vi "Ando Control.vi"() -> ()   [LabVIEW 2011]
panel:
  in  "Display Trace C":bool=TRUE
  in  "Trace C":enum16{"Fix", "Write"}(ring)=3
  in  "Display Trace B":bool=TRUE
  in  "Trace B":enum16{"Fix", "Write"}(ring)=3
  out "error out":errorcluster
  in  "Display Trace A":bool=TRUE
  in  "Trace A":enum16{"Fix", "Write"}(ring)=3
  in  "?":bool
  in  "?":bool
  in  "Log Scale dB/D (5)":dbl=10.0 min=0.1 max=10.0 step=0.1 format="%.1f"
  in  "Ref Level dBm (0)":dbl=-20.0 min=-90.0 max=20.0 step=0.1 format="%.1f"
  in  "Resolution (7: 2.0 nm)":T1(ring)
  in  "Sens (5:Norm Hold)":T2(ring)=enum."Norm Auto"
  in  "VISA session":refnum<visa-resource-name>="GPIB0::1::INSTR"
  in  "Span (1000 nm) 5":dbl=100.0 min=0.0 max=1200.0 step=0.1 format="%.2f"
  in  "Center (1250 nm) 5":dbl=1550.0 min=600.0 max=1750.0 step=0.01 format="%.2f"
  in  "Stop":bool
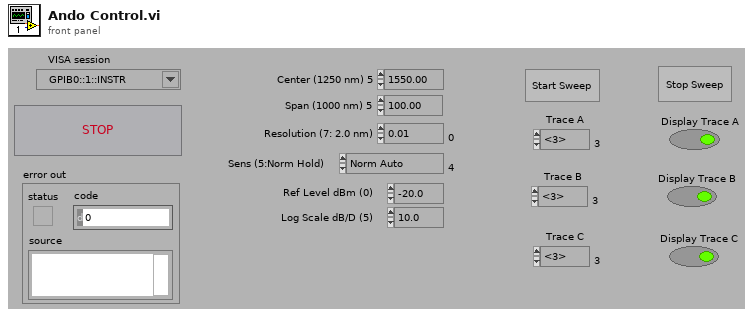
[diagram p1: front panel]
types:
  T1 = enum16{"0.01", "0.02", "0.05", "0.1", "0.2", "0.5", "1.0", "2.0"}
  T2 = enum16{"High 3", "High 2", "High 1", "Mid", "Norm Auto", "Norm Hold"}
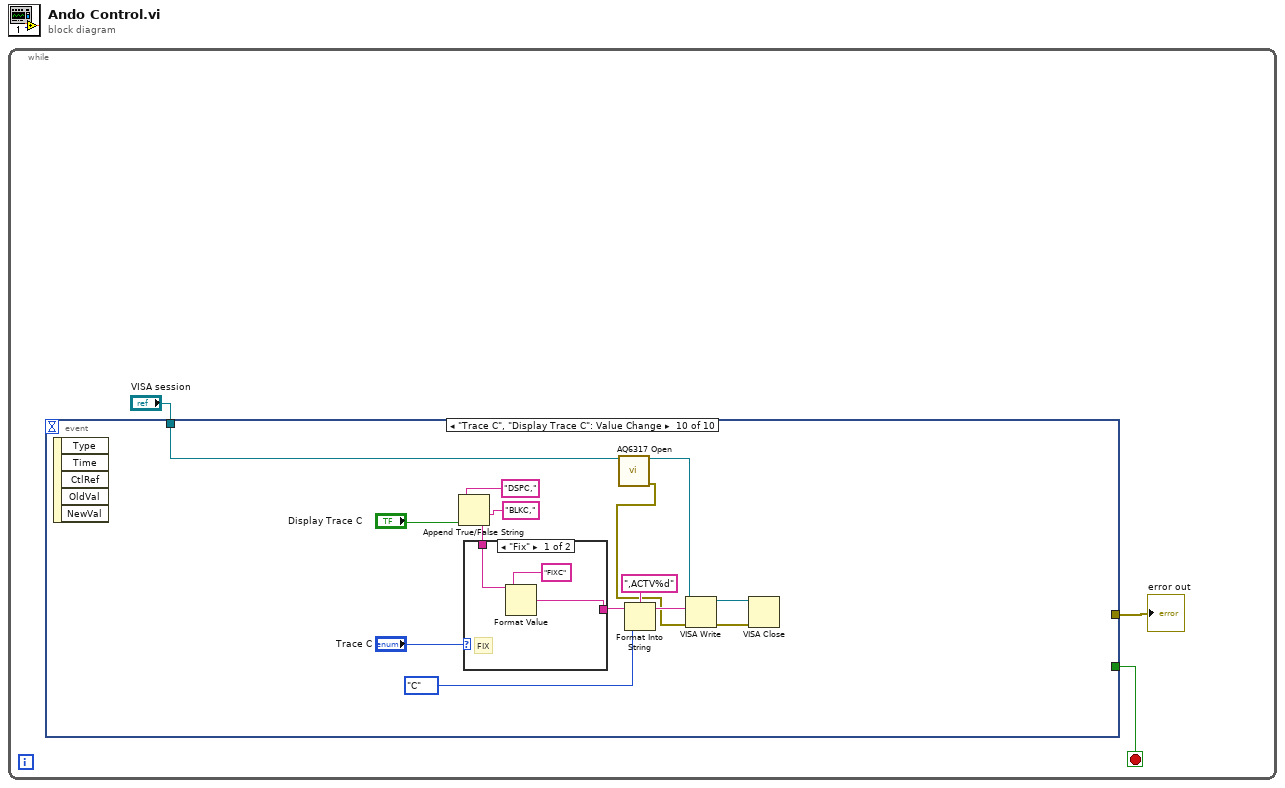
[diagram p0: block diagram]
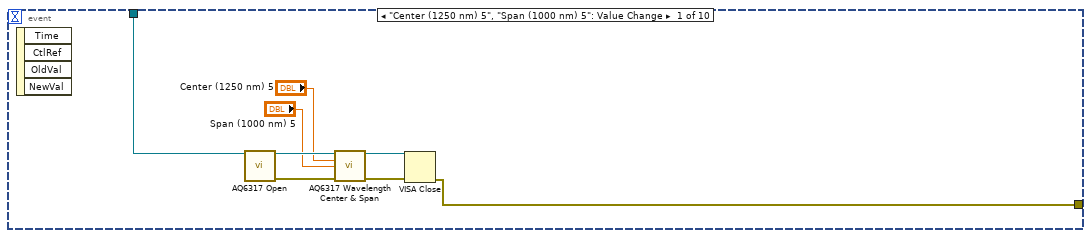
[diagram p2: hidden frame]
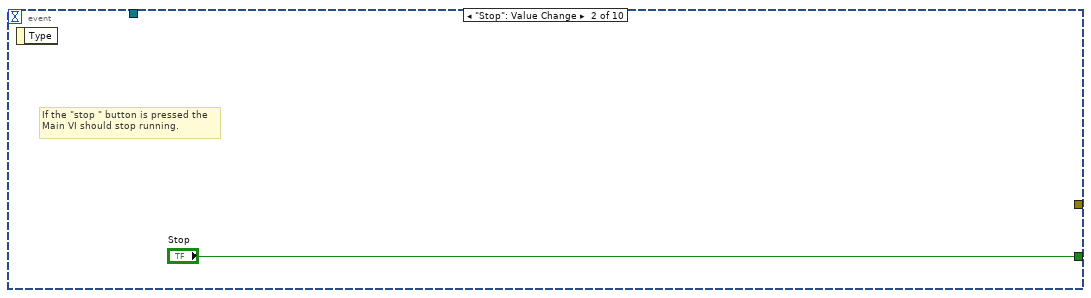
[diagram p3: hidden frame]
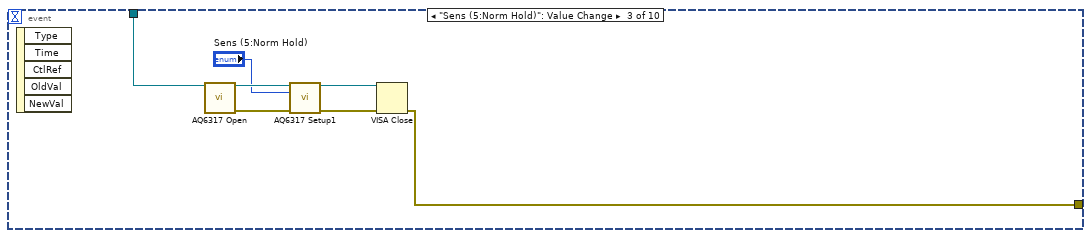
[diagram p4: hidden frame]
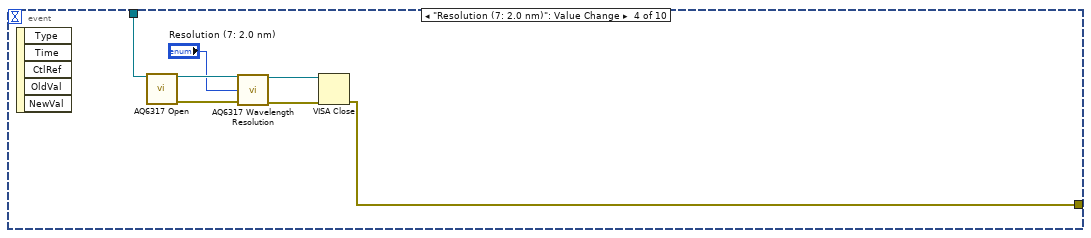
[diagram p5: hidden frame]
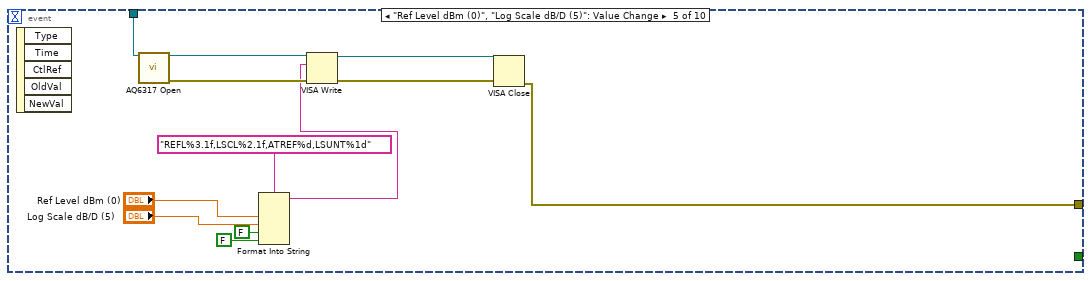
[diagram p6: hidden frame]
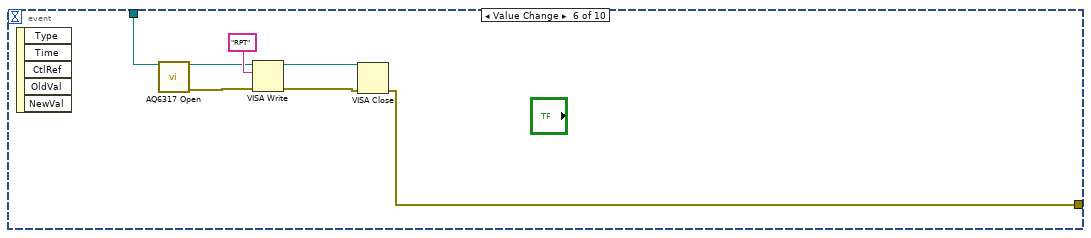
[diagram p7: hidden frame]
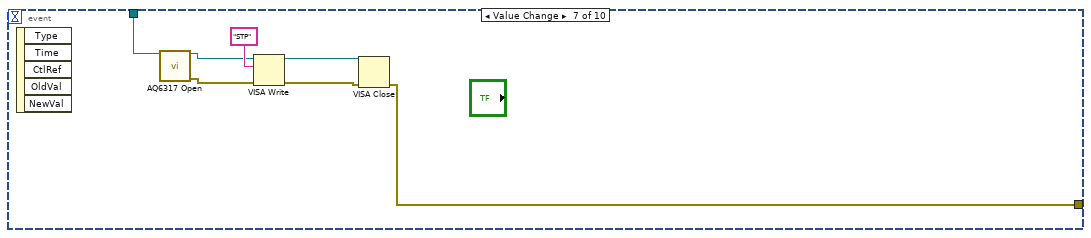
[diagram p8: hidden frame]
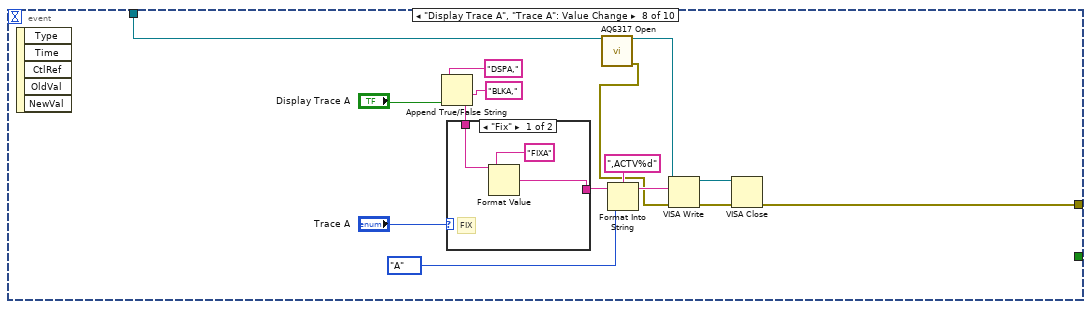
[diagram p9: hidden frame]
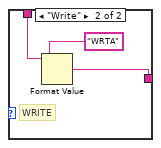
[diagram p10: hidden frame]
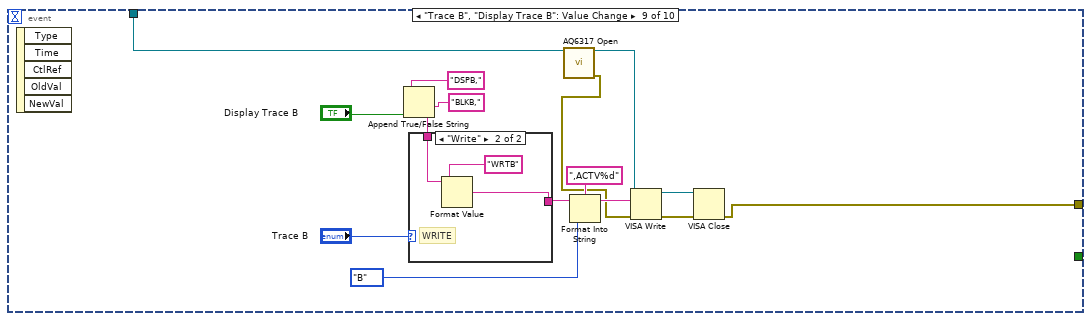
[diagram p11: hidden frame]
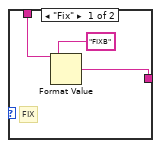
[diagram p12: hidden frame]
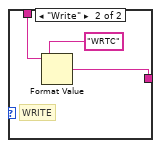
[diagram p13: hidden frame]
diagram:
  n1 = while {
    stop <- w3 stop-if-true
    n2 = event shown="[9] \"Trace C\", \"Display Trace C\": Value Change" {
      selector: _ -> [_ _ _ _ _ _ _ _ _ _]
      dyn-events: _ -> [_ _ _ _ _ _ _ _ _ _]
      timeout: _ -> [_ _ _ _ _ _ _ _ _ _]
      tunnel: [_ "Stop" _ _ _ _ _ _ _ _] -> w3
      tunnel: "VISA session" -> [w7 _ w19 w26 w36 w40 w51 w58 w75 w95]
      tunnel: [w4 _ w13 w20 w27 w39 w46 w53 w74 _] -> w1
      event "Center (1250 nm) 5", "Span (1000 nm) 5": Value Change {
        n3 = event-data() -> ()  [unwired: 5 out]
        n4 = call <instrlib>:"AQ6317 Open.vi"("VISA session (for class)"=w7) -> ("VISA session out"=w11:refnum<visa-resource-name>, "Error Out"=w10:errorcluster)  [unwired: 13 in]
        n5 = call <instrlib>:"AQ6317 Wavelength Center & Span.vi"("VISA session"=w11, "Center (1250 nm)"="Center (1250 nm) 5", "Span (1000 nm)"="Span (1000 nm) 5", "Error In"=w10) -> ("dup VISA session"=w9:refnum<visa-resource-name>, "Error Out"=w8:errorcluster)  [unwired: 10 in]
        n6 = VISA Close(VISA resource name=w9, error in (no error)=w8) -> (error out=w4:errorcluster)
      }
      event "Stop": Value Change {
        # "If the \"stop \" button is pressed the\nMain VI should stop running."
        n7 = event-data() -> ()  [unwired: 2 out]
      }
      event "Sens (5:Norm Hold)": Value Change {
        n8 = event-data() -> ()  [unwired: 6 out]
        n9 = call <instrlib>:"AQ6317 Open.vi"("VISA session (for class)"=w19) -> ("VISA session out"=w18:refnum<visa-resource-name>, "Error Out"=w17:errorcluster)  [unwired: 13 in]
        n10 = call <instrlib>:"AQ6317 Setup1.vi"("VISA session"=w18, "Sens (5:Norm Hold)"="Sens (5:Norm Hold)", "Error In"=w17) -> ("dup VISA session"=w15:refnum<visa-resource-name>, "Error Out"=w16:errorcluster)  [unwired: 11 in]
        n11 = VISA Close(VISA resource name=w15, error in (no error)=w16) -> (error out=w13:errorcluster)
      }
      event "Resolution (7: 2.0 nm)": Value Change {
        n12 = event-data() -> ()  [unwired: 6 out]
        n13 = call <instrlib>:"AQ6317 Open.vi"("VISA session (for class)"=w26) -> ("VISA session out"=w25:refnum<visa-resource-name>, "Error Out"=w23:errorcluster)  [unwired: 13 in]
        n14 = call <instrlib>:"AQ6317 Wavelength Resolution.vi"("VISA session"=w25, "Resolution (7: 2.0 nm)"="Resolution (7: 2.0 nm)", "Error In"=w23) -> ("dup VISA session"=w24:refnum<visa-resource-name>, "Error Out"=w22:errorcluster)  [unwired: 11 in]
        n15 = VISA Close(VISA resource name=w24, error in (no error)=w22) -> (error out=w20:errorcluster)
      }
      event "Ref Level dBm (0)", "Log Scale dB/D (5)": Value Change {
        n16 = event-data() -> ()  [unwired: 6 out]
        n17 = call <instrlib>:"AQ6317 Open.vi"("VISA session (for class)"=w36) -> ("VISA session out"=w35:refnum<visa-resource-name>, "Error Out"=w34:errorcluster)  [unwired: 13 in]
        n18 = Format Into String(format string="REFL%3.1f,LSCL%2.1f,ATREF%d,LSUNT%1d", "Ref Level dBm (0)", "Log Scale dB/D (5)", FALSE ("input 3"), FALSE ("input 4")) -> (resulting string=w28:string)  [unwired: 2 in, 1 out]
        n19 = VISA Write(VISA resource name=w35, write buffer=w28, error in (no error)=w34) -> (VISA resource name out=w37:refnum<visa-resource-name>, error out=w38:errorcluster)  [unwired: 1 out]
        n20 = VISA Close(VISA resource name=w37, error in (no error)=w38) -> (error out=w27:errorcluster)
      }
      event Value Change {
        n21 = event-data() -> ()  [unwired: 6 out]
        n22 = call <instrlib>:"AQ6317 Open.vi"("VISA session (for class)"=w40) -> ("VISA session out"=w44:refnum<visa-resource-name>, "Error Out"=w42:errorcluster)  [unwired: 13 in]
        n23 = VISA Write(VISA resource name=w44, write buffer="RPT", error in (no error)=w42) -> (VISA resource name out=w43:refnum<visa-resource-name>, error out=w41:errorcluster)  [unwired: 1 out]
        n24 = VISA Close(VISA resource name=w43, error in (no error)=w41) -> (error out=w39:errorcluster)
      }
      event Value Change {
        n25 = event-data() -> ()  [unwired: 6 out]
        n26 = call <instrlib>:"AQ6317 Open.vi"("VISA session (for class)"=w51) -> ("VISA session out"=w50:refnum<visa-resource-name>, "Error Out"=w48:errorcluster)  [unwired: 13 in]
        n27 = VISA Write(VISA resource name=w50, write buffer="STP", error in (no error)=w48) -> (VISA resource name out=w49:refnum<visa-resource-name>, error out=w47:errorcluster)  [unwired: 1 out]
        n28 = VISA Close(VISA resource name=w49, error in (no error)=w47) -> (error out=w46:errorcluster)
      }
      event "Display Trace A", "Trace A": Value Change {
        n29 = event-data() -> ()  [unwired: 6 out]
        n30 = Append True/False String(1:"Display Trace A", 2:"BLKA," ("false string"), 3:"DSPA," ("true string")) -> (0:w64:string)  [unwired: 1 in]
        n31 = case shown="\"Fix\"" "Trace A" {
          tunnel: w64 -> [w69 w72]
          tunnel: [w68 w71] -> w61
          frame "Fix" {
            # "FIX"
            n32 = Format Value(string ("")=w69, format string="FIXA") -> (output string=w68:string)  [unwired: 1 in]
          }
          frame "Write" {
            # "WRITE"
            n33 = Format Value(string ("")=w72, format string="WRTA") -> (output string=w71:string)  [unwired: 1 in]
          }
        }
        n34 = call <instrlib>:"AQ6317 Open.vi"("VISA session (for class)"=w58) -> ("VISA session out"=w57:refnum<visa-resource-name>, "Error Out"=w56:errorcluster)  [unwired: 13 in]
        n35 = Format Into String(format string=",ACTV%d", initial string=w61, enum16{"A", "B", "C"}."A" ("Active Trace (0:A)")) -> (resulting string=w60:string)  [unwired: 1 in, 1 out]
        n36 = VISA Write(VISA resource name=w57, write buffer=w60, error in (no error)=w56) -> (VISA resource name out=w55:refnum<visa-resource-name>, error out=w54:errorcluster)  [unwired: 1 out]
        n37 = VISA Close(VISA resource name=w55, error in (no error)=w54) -> (error out=w53:errorcluster)
      }
      event "Trace B", "Display Trace B": Value Change {
        n38 = event-data() -> ()  [unwired: 6 out]
        n39 = Append True/False String(1:"Display Trace B", 2:"BLKB," ("false string"), 3:"DSPB," ("true string")) -> (0:w85:string)  [unwired: 1 in]
        n40 = case shown="\"Write\"" "Trace B" {
          tunnel: w85 -> [w90 w93]
          tunnel: [w89 w92] -> w82
          frame "Fix" {
            # "FIX"
            n41 = Format Value(string ("")=w90, format string="FIXB") -> (output string=w89:string)  [unwired: 1 in]
          }
          frame "Write" {
            # "WRITE"
            n42 = Format Value(string ("")=w93, format string="WRTB") -> (output string=w92:string)  [unwired: 1 in]
          }
        }
        n43 = call <instrlib>:"AQ6317 Open.vi"("VISA session (for class)"=w75) -> ("VISA session out"=w79:refnum<visa-resource-name>, "Error Out"=w78:errorcluster)  [unwired: 13 in]
        n44 = Format Into String(format string=",ACTV%d", initial string=w82, enum16{"A", "B", "C"}."B" ("Active Trace (0:A)")) -> (resulting string=w81:string)  [unwired: 1 in, 1 out]
        n45 = VISA Write(VISA resource name=w79, write buffer=w81, error in (no error)=w78) -> (VISA resource name out=w77:refnum<visa-resource-name>, error out=w76:errorcluster)  [unwired: 1 out]
        n46 = VISA Close(VISA resource name=w77, error in (no error)=w76) -> (error out=w74:errorcluster)
      }
      event "Trace C", "Display Trace C": Value Change {
        n47 = event-data() -> ()  [unwired: 6 out]
        n48 = Append True/False String(1:"Display Trace C", 2:"BLKC," ("false string"), 3:"DSPC," ("true string")) -> (0:w105:string)  [unwired: 1 in]
        n49 = case shown="\"Fix\"" "Trace C" {
          tunnel: w105 -> [w110 w113]
          tunnel: [w109 w112] -> w102
          frame "Fix" {
            # "FIX"
            n50 = Format Value(string ("")=w110, format string="FIXC") -> (output string=w109:string)  [unwired: 1 in]
          }
          frame "Write" {
            # "WRITE"
            n51 = Format Value(string ("")=w113, format string="WRTC") -> (output string=w112:string)  [unwired: 1 in]
          }
        }
        n52 = call <instrlib>:"AQ6317 Open.vi"("VISA session (for class)"=w95) -> ("VISA session out"=w99:refnum<visa-resource-name>, "Error Out"=w98:errorcluster)  [unwired: 13 in]
        n53 = Format Into String(format string=",ACTV%d", initial string=w102, enum16{"A", "B", "C"}."C" ("Active Trace (0:A)")) -> (resulting string=w101:string)  [unwired: 1 in, 1 out]
        n54 = VISA Write(VISA resource name=w99, write buffer=w101, error in (no error)=w98) -> (VISA resource name out=w97:refnum<visa-resource-name>, error out=w96:errorcluster)  [unwired: 1 out]
        n55 = VISA Close(VISA resource name=w97, error in (no error)=w96) -> ()  [unwired: 1 out]
      }
    }
    "error out" <- w1
  }
